vi "Yellow 1 to 2_spacial.vi"   [LabVIEW 2019]
uses:
  Global Var.vi
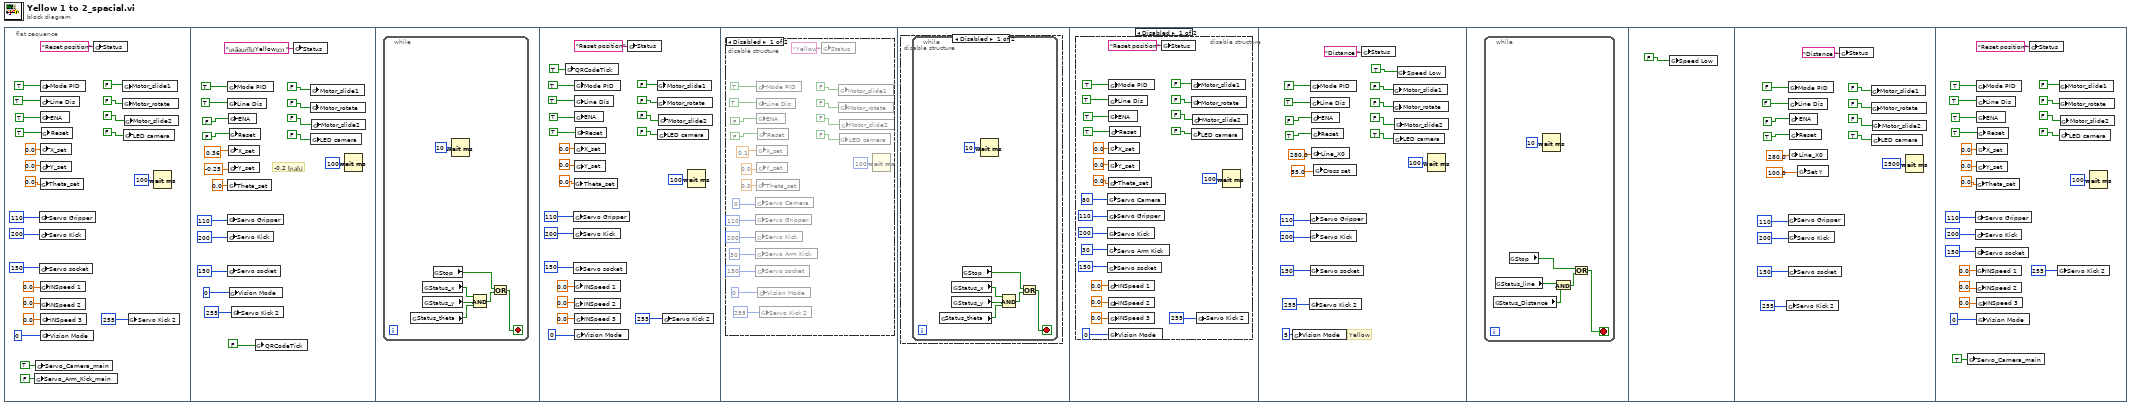
[diagram p0: block diagram]
diagram:
  n1 = flat-sequence {
    frame #0 {
      n2 = global write "Global Var.vi" "Servo_Arm_Kick_main"(FALSE ("Mode PID")) -> ()
      n3 = global write "Global Var.vi" "Servo_Camera_main"(TRUE ("Mode PID")) -> ()
      n4 = global write "Global Var.vi" "Servo Gripper"(u8 110 ("Servo Camera")) -> ()
      n5 = global write "Global Var.vi" "Servo Kick"(u8 200 ("Servo Camera")) -> ()
      n6 = global write "Global Var.vi" "Servo socket"(u8 150 ("Servo Camera")) -> ()
      n7 = global write "Global Var.vi" "Theta_set"(0.0 ("Theta_set")) -> ()
      n8 = global write "Global Var.vi" "INSpeed 1"(0.0 ("X_set")) -> ()
      n9 = global write "Global Var.vi" "INSpeed 2"(0.0 ("Y_set")) -> ()
      n10 = global write "Global Var.vi" "Mode PID"(TRUE ("Mode PID")) -> ()
      n11 = global write "Global Var.vi" "Line Dis"(TRUE ("Mode PID")) -> ()
      n12 = global write "Global Var.vi" "ENA"(TRUE ("ENA")) -> ()
      n13 = global write "Global Var.vi" "X_set"(0.0 ("X_set")) -> ()
      n14 = global write "Global Var.vi" "Y_set"(0.0 ("Y_set")) -> ()
      n15 = global write "Global Var.vi" "INSpeed 3"(0.0 ("Theta_set")) -> ()
      n16 = global write "Global Var.vi" "Vision Mode"(i16 0 ("Vision Mode")) -> ()
      n17 = global write "Global Var.vi" "Reset"(TRUE ("ENA")) -> ()
      n18 = global write "Global Var.vi" "Status"("Reset position" ("Status")) -> ()
      n19 = global write "Global Var.vi" "Motor_slide1"(FALSE ("Mode PID")) -> ()
      n20 = global write "Global Var.vi" "Motor_rotate"(FALSE ("ENA")) -> ()
      n21 = global write "Global Var.vi" "LED camera"(FALSE ("LED camera")) -> ()
      n22 = global write "Global Var.vi" "Motor_slide2"(FALSE ("ENA")) -> ()
      n23 = global write "Global Var.vi" "Servo Kick 2"(u8 255 ("Servo Camera")) -> ()
      n24 = Wait (ms)(milliseconds to wait=u32 100) -> ()  [unwired: 1 out]
    }
    frame #1 {
      # "-0.2 ไกลไป"
      n25 = global write "Global Var.vi" "Servo Gripper"(u8 110 ("Servo Camera")) -> ()
      n26 = global write "Global Var.vi" "Servo Kick"(u8 200 ("Servo Camera")) -> ()
      n27 = global write "Global Var.vi" "Servo socket"(u8 150 ("Servo Camera")) -> ()
      n28 = global write "Global Var.vi" "Mode PID"(TRUE ("Mode PID")) -> ()
      n29 = global write "Global Var.vi" "Line Dis"(TRUE ("Mode PID")) -> ()
      n30 = global write "Global Var.vi" "Theta_set"(0.0 ("Theta_set")) -> ()
      n31 = global write "Global Var.vi" "ENA"(FALSE ("ENA")) -> ()
      n32 = global write "Global Var.vi" "X_set"(0.36 ("X_set")) -> ()
      n33 = global write "Global Var.vi" "Y_set"(-0.25 ("Y_set")) -> ()
      n34 = global write "Global Var.vi" "Reset"(FALSE ("ENA")) -> ()
      n35 = global write "Global Var.vi" "Vision Mode"(i16 0 ("Vision Mode")) -> ()
      n36 = global write "Global Var.vi" "Servo Kick 2"(u8 255 ("Servo Camera")) -> ()
      n37 = global write "Global Var.vi" "QRCodeTick"(FALSE ("ENA")) -> ()
      n38 = global write "Global Var.vi" "Status"("เคลื่อนที่ไปYellowขวา " ("Status")) -> ()
      n39 = global write "Global Var.vi" "Motor_slide1"(FALSE ("Mode PID")) -> ()
      n40 = global write "Global Var.vi" "Motor_rotate"(FALSE ("ENA")) -> ()
      n41 = global write "Global Var.vi" "LED camera"(FALSE ("LED camera")) -> ()
      n42 = global write "Global Var.vi" "Motor_slide2"(FALSE ("ENA")) -> ()
      n43 = Wait (ms)(milliseconds to wait=u32 100) -> ()  [unwired: 1 out]
    }
    frame #2 {
      n44 = while {
        stop <- w45 stop-if-true
        n45 = global read "Global Var.vi" "Status_theta"() -> (w47:bool)
        n46 = global read "Global Var.vi" "Status_x"() -> (w48:bool)
        n47 = global read "Global Var.vi" "Status_y"() -> (w49:bool)
        n48 = global read "Global Var.vi" "Stop"() -> (w43:bool)
        n49 = Wait (ms)(milliseconds to wait=u32 10) -> ()  [unwired: 1 out]
        n50 = Compound Arithmetic op=AND(w48, w49, w47) -> (w44:bool)
        n51 = Or(x=w43, y=w44) -> (x .or. y?=w45:bool)
      }
    }
    frame #3 {
      n52 = global write "Global Var.vi" "QRCodeTick"(TRUE ("ENA")) -> ()
      n53 = global write "Global Var.vi" "Servo Gripper"(u8 110 ("Servo Camera")) -> ()
      n54 = global write "Global Var.vi" "Servo Kick"(u8 200 ("Servo Camera")) -> ()
      n55 = global write "Global Var.vi" "Servo socket"(u8 150 ("Servo Camera")) -> ()
      n56 = global write "Global Var.vi" "Theta_set"(0.0 ("Theta_set")) -> ()
      n57 = global write "Global Var.vi" "INSpeed 1"(0.0 ("X_set")) -> ()
      n58 = global write "Global Var.vi" "INSpeed 2"(0.0 ("Y_set")) -> ()
      n59 = global write "Global Var.vi" "Mode PID"(TRUE ("Mode PID")) -> ()
      n60 = global write "Global Var.vi" "Line Dis"(TRUE ("Mode PID")) -> ()
      n61 = global write "Global Var.vi" "ENA"(TRUE ("ENA")) -> ()
      n62 = global write "Global Var.vi" "X_set"(0.0 ("X_set")) -> ()
      n63 = global write "Global Var.vi" "Y_set"(0.0 ("Y_set")) -> ()
      n64 = global write "Global Var.vi" "INSpeed 3"(0.0 ("Theta_set")) -> ()
      n65 = global write "Global Var.vi" "Vision Mode"(i16 0 ("Vision Mode")) -> ()
      n66 = global write "Global Var.vi" "Reset"(TRUE ("ENA")) -> ()
      n67 = global write "Global Var.vi" "Status"("Reset position" ("Status")) -> ()
      n68 = global write "Global Var.vi" "Motor_slide1"(FALSE ("Mode PID")) -> ()
      n69 = global write "Global Var.vi" "Motor_rotate"(FALSE ("ENA")) -> ()
      n70 = global write "Global Var.vi" "LED camera"(FALSE ("LED camera")) -> ()
      n71 = global write "Global Var.vi" "Motor_slide2"(FALSE ("ENA")) -> ()
      n72 = global write "Global Var.vi" "Servo Kick 2"(u8 255 ("Servo Camera")) -> ()
      n73 = Wait (ms)(milliseconds to wait=u32 100) -> ()  [unwired: 1 out]
    }
    frame #4 {
      n74 = disable-structure shown="Disabled" {
        frame Disabled {
          n75 = global write "Global Var.vi" "Servo Camera"(u8 0 ("Servo Camera")) -> ()
          n76 = global write "Global Var.vi" "Servo Gripper"(u8 110 ("Servo Camera")) -> ()
          n77 = global write "Global Var.vi" "Servo Kick"(u8 200 ("Servo Camera")) -> ()
          n78 = global write "Global Var.vi" "Servo Arm Kick"(u8 30 ("Servo Camera")) -> ()
          n79 = global write "Global Var.vi" "Servo socket"(u8 150 ("Servo Camera")) -> ()
          n80 = global write "Global Var.vi" "Mode PID"(TRUE ("Mode PID")) -> ()
          n81 = global write "Global Var.vi" "Line Dis"(TRUE ("Mode PID")) -> ()
          n82 = global write "Global Var.vi" "Theta_set"(0.0 ("Theta_set")) -> ()
          n83 = global write "Global Var.vi" "ENA"(FALSE ("ENA")) -> ()
          n84 = global write "Global Var.vi" "X_set"(0.1 ("X_set")) -> ()
          n85 = global write "Global Var.vi" "Y_set"(0.0 ("Y_set")) -> ()
          n86 = global write "Global Var.vi" "Reset"(FALSE ("ENA")) -> ()
          n87 = global write "Global Var.vi" "Vision Mode"(i16 0 ("Vision Mode")) -> ()
          n88 = global write "Global Var.vi" "Servo Kick 2"(u8 255 ("Servo Camera")) -> ()
          n89 = global write "Global Var.vi" "Status"("Yellow" ("Status")) -> ()
          n90 = global write "Global Var.vi" "Motor_slide1"(FALSE ("Mode PID")) -> ()
          n91 = global write "Global Var.vi" "Motor_rotate"(FALSE ("ENA")) -> ()
          n92 = global write "Global Var.vi" "LED camera"(FALSE ("LED camera")) -> ()
          n93 = global write "Global Var.vi" "Motor_slide2"(FALSE ("ENA")) -> ()
          n94 = Wait (ms)(milliseconds to wait=u32 100) -> ()  [unwired: 1 out]
        }
        frame Enabled {
        }
      }
    }
    frame #5 {
      n95 = disable-structure shown="Disabled" {
        frame Disabled {
          n96 = while {
            stop <- w94 stop-if-true
            n97 = global read "Global Var.vi" "Status_theta"() -> (w96:bool)
            n98 = global read "Global Var.vi" "Status_x"() -> (w97:bool)
            n99 = global read "Global Var.vi" "Status_y"() -> (w98:bool)
            n100 = global read "Global Var.vi" "Stop"() -> (w92:bool)
            n101 = Wait (ms)(milliseconds to wait=u32 10) -> ()  [unwired: 1 out]
            n102 = Compound Arithmetic op=AND(w97, w98, w96) -> (w93:bool)
            n103 = Or(x=w92, y=w93) -> (x .or. y?=w94:bool)
          }
        }
        frame Enabled {
        }
      }
    }
    frame #6 {
      n104 = disable-structure shown="Disabled" {
        frame Disabled {
          n105 = global write "Global Var.vi" "Servo Camera"(u8 80 ("Servo Camera")) -> ()
          n106 = global write "Global Var.vi" "Servo Gripper"(u8 110 ("Servo Camera")) -> ()
          n107 = global write "Global Var.vi" "Servo Kick"(u8 200 ("Servo Camera")) -> ()
          n108 = global write "Global Var.vi" "Servo Arm Kick"(u8 30 ("Servo Camera")) -> ()
          n109 = global write "Global Var.vi" "Servo socket"(u8 150 ("Servo Camera")) -> ()
          n110 = global write "Global Var.vi" "Theta_set"(0.0 ("Theta_set")) -> ()
          n111 = global write "Global Var.vi" "INSpeed 1"(0.0 ("X_set")) -> ()
          n112 = global write "Global Var.vi" "INSpeed 2"(0.0 ("Y_set")) -> ()
          n113 = global write "Global Var.vi" "Mode PID"(TRUE ("Mode PID")) -> ()
          n114 = global write "Global Var.vi" "Line Dis"(TRUE ("Mode PID")) -> ()
          n115 = global write "Global Var.vi" "ENA"(TRUE ("ENA")) -> ()
          n116 = global write "Global Var.vi" "X_set"(0.0 ("X_set")) -> ()
          n117 = global write "Global Var.vi" "Y_set"(0.0 ("Y_set")) -> ()
          n118 = global write "Global Var.vi" "INSpeed 3"(0.0 ("Theta_set")) -> ()
          n119 = global write "Global Var.vi" "Vision Mode"(i16 0 ("Vision Mode")) -> ()
          n120 = global write "Global Var.vi" "Reset"(TRUE ("ENA")) -> ()
          n121 = global write "Global Var.vi" "Status"("Reset position" ("Status")) -> ()
          n122 = global write "Global Var.vi" "Motor_slide1"(FALSE ("Mode PID")) -> ()
          n123 = global write "Global Var.vi" "Motor_rotate"(FALSE ("ENA")) -> ()
          n124 = global write "Global Var.vi" "LED camera"(FALSE ("LED camera")) -> ()
          n125 = global write "Global Var.vi" "Motor_slide2"(FALSE ("ENA")) -> ()
          n126 = global write "Global Var.vi" "Servo Kick 2"(u8 255 ("Servo Camera")) -> ()
          n127 = Wait (ms)(milliseconds to wait=u32 100) -> ()  [unwired: 1 out]
        }
        frame Enabled {
        }
      }
    }
    frame #7 {
      # "Yellow"
      n128 = global write "Global Var.vi" "Vision Mode"(i16 5 ("Vision Mode")) -> ()
      n129 = global write "Global Var.vi" "Servo Kick 2"(u8 255 ("Servo Camera")) -> ()
      n130 = global write "Global Var.vi" "Servo Gripper"(u8 110 ("Servo Camera")) -> ()
      n131 = global write "Global Var.vi" "Servo Kick"(u8 200 ("Servo Camera")) -> ()
      n132 = global write "Global Var.vi" "Servo socket"(u8 150 ("Servo Camera")) -> ()
      n133 = global write "Global Var.vi" "Mode PID"(FALSE ("Mode PID")) -> ()
      n134 = global write "Global Var.vi" "Line Dis"(TRUE ("Mode PID")) -> ()
      n135 = global write "Global Var.vi" "ENA"(FALSE ("ENA")) -> ()
      n136 = global write "Global Var.vi" "Line_X0"(280.0 ("Y_set")) -> ()
      n137 = global write "Global Var.vi" "Reset"(TRUE ("ENA")) -> ()
      n138 = global write "Global Var.vi" "Cross set"(55.0 ("Y_set")) -> ()
      n139 = global write "Global Var.vi" "Status"("Distance " ("Status")) -> ()
      n140 = global write "Global Var.vi" "Motor_slide1"(FALSE ("Mode PID")) -> ()
      n141 = global write "Global Var.vi" "Motor_rotate"(FALSE ("ENA")) -> ()
      n142 = global write "Global Var.vi" "LED camera"(TRUE ("LED camera")) -> ()
      n143 = global write "Global Var.vi" "Motor_slide2"(FALSE ("ENA")) -> ()
      n144 = global write "Global Var.vi" "Speed Low"(TRUE ("Mode PID")) -> ()
      n145 = Wait (ms)(milliseconds to wait=u32 100) -> ()  [unwired: 1 out]
    }
    frame #8 {
      n146 = while {
        stop <- w144 stop-if-true
        n147 = global read "Global Var.vi" "Status_Distance"() -> (w140:bool)
        n148 = global read "Global Var.vi" "Status_line"() -> (w141:bool)
        n149 = global read "Global Var.vi" "Stop"() -> (w143:bool)
        n150 = Wait (ms)(milliseconds to wait=u32 10) -> ()  [unwired: 1 out]
        n151 = And(x=w141, y=w140) -> (x .and. y?=w142:bool)
        n152 = Or(x=w143, y=w142) -> (x .or. y?=w144:bool)
      }
    }
    frame #9 {
      n153 = global write "Global Var.vi" "Speed Low"(FALSE ("Mode PID")) -> ()
    }
    frame #10 {
      n154 = global write "Global Var.vi" "Servo Kick 2"(u8 255 ("Servo Camera")) -> ()
      n155 = global write "Global Var.vi" "Servo Gripper"(u8 110 ("Servo Camera")) -> ()
      n156 = global write "Global Var.vi" "Servo Kick"(u8 200 ("Servo Camera")) -> ()
      n157 = global write "Global Var.vi" "Servo socket"(u8 150 ("Servo Camera")) -> ()
      n158 = global write "Global Var.vi" "Mode PID"(FALSE ("Mode PID")) -> ()
      n159 = global write "Global Var.vi" "Line Dis"(FALSE ("Mode PID")) -> ()
      n160 = global write "Global Var.vi" "ENA"(FALSE ("ENA")) -> ()
      n161 = global write "Global Var.vi" "Line_X0"(280.0 ("Y_set")) -> ()
      n162 = global write "Global Var.vi" "Reset"(TRUE ("ENA")) -> ()
      n163 = global write "Global Var.vi" "Set Y"(100.0 ("Y_set")) -> ()
      n164 = global write "Global Var.vi" "Status"("Distance " ("Status")) -> ()
      n165 = global write "Global Var.vi" "Motor_slide1"(FALSE ("Mode PID")) -> ()
      n166 = global write "Global Var.vi" "Motor_rotate"(FALSE ("ENA")) -> ()
      n167 = global write "Global Var.vi" "LED camera"(TRUE ("LED camera")) -> ()
      n168 = global write "Global Var.vi" "Motor_slide2"(FALSE ("ENA")) -> ()
      n169 = Wait (ms)(milliseconds to wait=u32 2500) -> ()  [unwired: 1 out]
    }
    frame #11 {
      n170 = global write "Global Var.vi" "Servo_Camera_main"(TRUE ("Mode PID")) -> ()
      n171 = global write "Global Var.vi" "Servo Gripper"(u8 110 ("Servo Camera")) -> ()
      n172 = global write "Global Var.vi" "Servo Kick"(u8 200 ("Servo Camera")) -> ()
      n173 = global write "Global Var.vi" "Servo socket"(u8 150 ("Servo Camera")) -> ()
      n174 = global write "Global Var.vi" "Theta_set"(0.0 ("Theta_set")) -> ()
      n175 = global write "Global Var.vi" "INSpeed 1"(0.0 ("X_set")) -> ()
      n176 = global write "Global Var.vi" "INSpeed 2"(0.0 ("Y_set")) -> ()
      n177 = global write "Global Var.vi" "Mode PID"(TRUE ("Mode PID")) -> ()
      n178 = global write "Global Var.vi" "Line Dis"(TRUE ("Mode PID")) -> ()
      n179 = global write "Global Var.vi" "ENA"(TRUE ("ENA")) -> ()
      n180 = global write "Global Var.vi" "X_set"(0.0 ("X_set")) -> ()
      n181 = global write "Global Var.vi" "Y_set"(0.0 ("Y_set")) -> ()
      n182 = global write "Global Var.vi" "INSpeed 3"(0.0 ("Theta_set")) -> ()
      n183 = global write "Global Var.vi" "Vision Mode"(i16 0 ("Vision Mode")) -> ()
      n184 = global write "Global Var.vi" "Reset"(TRUE ("ENA")) -> ()
      n185 = global write "Global Var.vi" "Status"("Reset position" ("Status")) -> ()
      n186 = global write "Global Var.vi" "Servo Kick 2"(u8 255 ("Servo Camera")) -> ()
      n187 = global write "Global Var.vi" "Motor_slide1"(FALSE ("Mode PID")) -> ()
      n188 = global write "Global Var.vi" "Motor_rotate"(FALSE ("ENA")) -> ()
      n189 = global write "Global Var.vi" "LED camera"(FALSE ("LED camera")) -> ()
      n190 = global write "Global Var.vi" "Motor_slide2"(FALSE ("ENA")) -> ()
      n191 = Wait (ms)(milliseconds to wait=u32 100) -> ()  [unwired: 1 out]
    }
  }
